vi "WoD Main.vi"() -> ()   [LabVIEW 2017]
uses:
  <vilib>/Platform/TimedLoop/XDataNode/wakeup.ctl
  <vilib>/Platform/TimedLoop/XDataNode/XDNodeRunTimeDep.lvlib
  <vilib>/Platform/TimedLoop/XDataNode/nitl_modes.ctl
  <vilib>/Platform/TimedLoop/XDataNode/timing_clust.ctl
  <vilib>/platform/TimedLoop/XDataNode/XDataNode.xnode
  <vilib>/myRIO/Common/Instrument Driver Framework/myRIO v1.0/DIO/typedefs/DIO Channels Enum.ctl
  <vilib>/myRIO/Common/Instrument Driver Framework/myRIO v1.0/DIO/typedefs/DIO Channels List.ctl
  <vilib>/myRIO/Common/Instrument Driver Framework/Utilities/typedefs/Generic FPGA Reference.ctl
  <vilib>/myRIO/Common/Instrument Driver Framework/Utilities/typedefs/myRIO v1.0 Reference.ctl
  <vilib>/myRIO/Common/Instrument Driver Framework/Utilities/typedefs/Hardware Version Enum.ctl
  <vilib>/myRIO/Common/Instrument Driver Framework/Utilities/typedefs/myRIO Generic Hardware Reference.ctl
  <vilib>/myRIO/Instrument Drivers/Onboard IO/DIO/typedefs/DIO Reference.ctl
  <vilib>/myRIO/Instrument Drivers/Onboard IO/DIO/DIO.lvlib
  <vilib>/myRIO/Instrument Drivers/Onboard IO/DIO/vis/Read.vi
  <vilib>/myRIO/Instrument Drivers/Onboard IO/DIO/vis/myRIO DIO Open.xnode
  <vilib>/myRIO/Common/Instrument Driver Framework/Utilities/vis/Is FPGA Ref Available.vi
  <vilib>/myRIO/Express VI/Onboard IO/DI/DI Express VI.xnode
  <vilib>/myRIO/Common/Instrument Driver Framework/myRIO v1.0/DIO/vis/myRIO v1.1 Open DIO.vi
  <vilib>/userdefined/High Color/nirio_resource_hc.ctl
panel:
  out "Laser Error":errorcluster
  in  "Stop Button":bool
  in  "Select Test":T1(ring)
  in  "Air Bearings?":bool
  in  "Target Speed (rpm)":u32
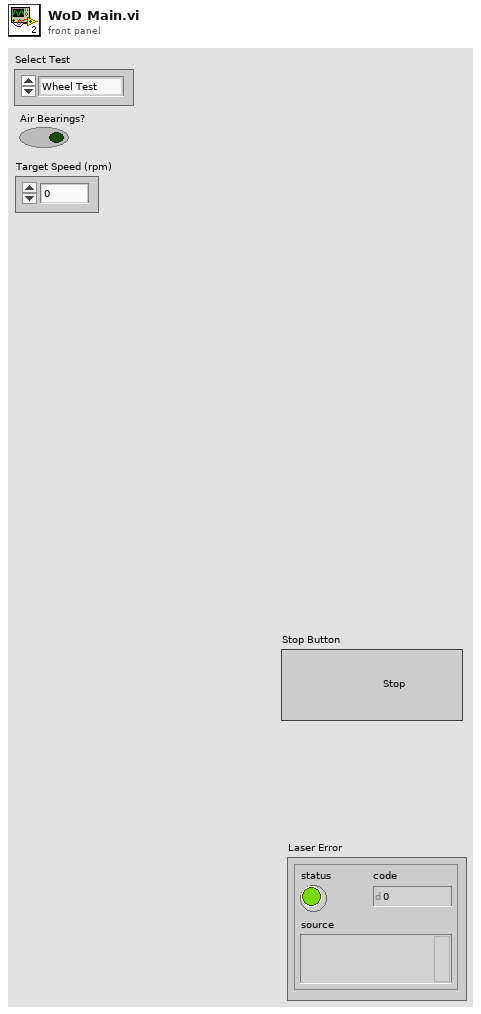
[diagram p1: front panel]
types:
  T1 = enum16{"Wheel Test", "Magnetic Braking Test", "Friction Brake Test", "Material Test", "Air Bearing Test"}
  T2 = typedef "XDNodeRunTimeDep.lvlib/timing_clust.ctl" = cluster{"Expected End [f-1]":u64, "Actual End [f-1]":u64, "Finished Late? [f-1]":bool, "Expected End [i-1]":u64, "Actual End [i-1]":u64, "Finished Late? [i-1]":bool, "Expected Start [i]":u64, "Actual Start [i]":u64, "Expected Start [f]":u64, "Actual Start [f]":u64, "Source Name":string, "Structure Name":string, "Period":i64, "Deadline":i64, "Offset":i64, "Start":i64, "Priority":i32, "Timeout":i32, "Mode":T3, "Wakeup Reason":T4, "Error":errorcluster, "Source Type":string, "Secondary Source Type":string, "Global End Time":u64, "Global Start Time":u64, "Frame Duration":u64, "Iteration Duration":u64, "Assigned CPU":i32, "I/O Scan Engine Mode":u32}
  T3 = typedef "XDNodeRunTimeDep.lvlib/nitl_modes.ctl" = enum32{"No Change", "Process missed periods, maintain original phase", "Discard missed periods, maintain original phase", "Process missed periods, ignore original phase", "Discard missed periods, ignore original phase"}
  T4 = typedef "XDNodeRunTimeDep.lvlib/wakeup.ctl" = enum32{"Normal", "Aborted", "Asynchronous wakeup", "Timing source error", "Timed loop error", "Timeout"}
  T5 = typedef "DIO.lvlib/DIO Reference.ctl" = cluster{"myRIO Reference":T6, "DIO Channels List":T10}
  T6 = typedef "myRIO Generic Hardware Reference.ctl" = cluster{"myRIO Model":T7, "myRIO Hardware Reference":T8}
  T7 = typedef "Hardware Version Enum.ctl" = enum16{"Unknown", "myRIO-1900", "myRIO-1950", "roboRIO", "NI ELVIS RIO CM"}
  T8 = typedef "myRIO v1.0 Reference.ctl" = cluster{"Generic FPGA Reference":T9, "Allow multiple opens":bool}
  T9 = typedef "Generic FPGA Reference.ctl" = refnum<k20>
  T10 = typedef "DIO Channels List.ctl" = T11[]
  T11 = typedef "DIO Channels Enum.ctl" = enum16{"Not Connected", "C/DIO0", "C/DIO1", "C/DIO2", "C/DIO3", "C/DIO4", "C/DIO5", "C/DIO6", "C/DIO7", "A/DIO0", "A/DIO1", "A/DIO2", "A/DIO3", "A/DIO4", "A/DIO5", "A/DIO6", "A/DIO7", "A/DIO8", "A/DIO9", "A/DIO10", "A/DIO11", "A/DIO12", "A/DIO13", "A/DIO14", "A/DIO15", "B/DIO0", "B/DIO1", "B/DIO2", "B/DIO3", "B/DIO4", "B/DIO5", "B/DIO6", "B/DIO7", "B/DIO8", "B/DIO9", "B/DIO10", "B/DIO11", "B/DIO12", "B/DIO13", "B/DIO14", "B/DIO15", "LED0", "LED1", "LED2", "LED3", "Button0", "DIO/DIO0", "DIO/DIO1", "DIO/DIO2", "DIO/DIO3", "DIO/DIO4", "DIO/DIO5", "DIO/DIO6", "DIO/DIO7", "DIO/DIO8", "DIO/DIO9", "SPI/CS0", "SPI/CS1", "SPI/CS2", "SPI/CS3", "LED RADIO (Green)", "LED RADIO (Red)", "LED COMM (Green)", "LED COMM (Red)", "LED MODE (Green)", "LED MODE (Red)"}
  T12 = typedef "nirio_resource_hc.ctl" = tag
  T13 = typedef "allLaserReadings.ctl" = cluster{"Fancy Laser 1":T14, "Fancy Laser 2":T14, "Simple Laser 1":T14, "Simple Laser 2":T14, "Time Stamp":timestamp}
  T14 = typedef "laserReading.ctl" = cluster{"Laser":bool, "Stripe Count":u32, "Last 10 Rising Edges":timestamp[]}
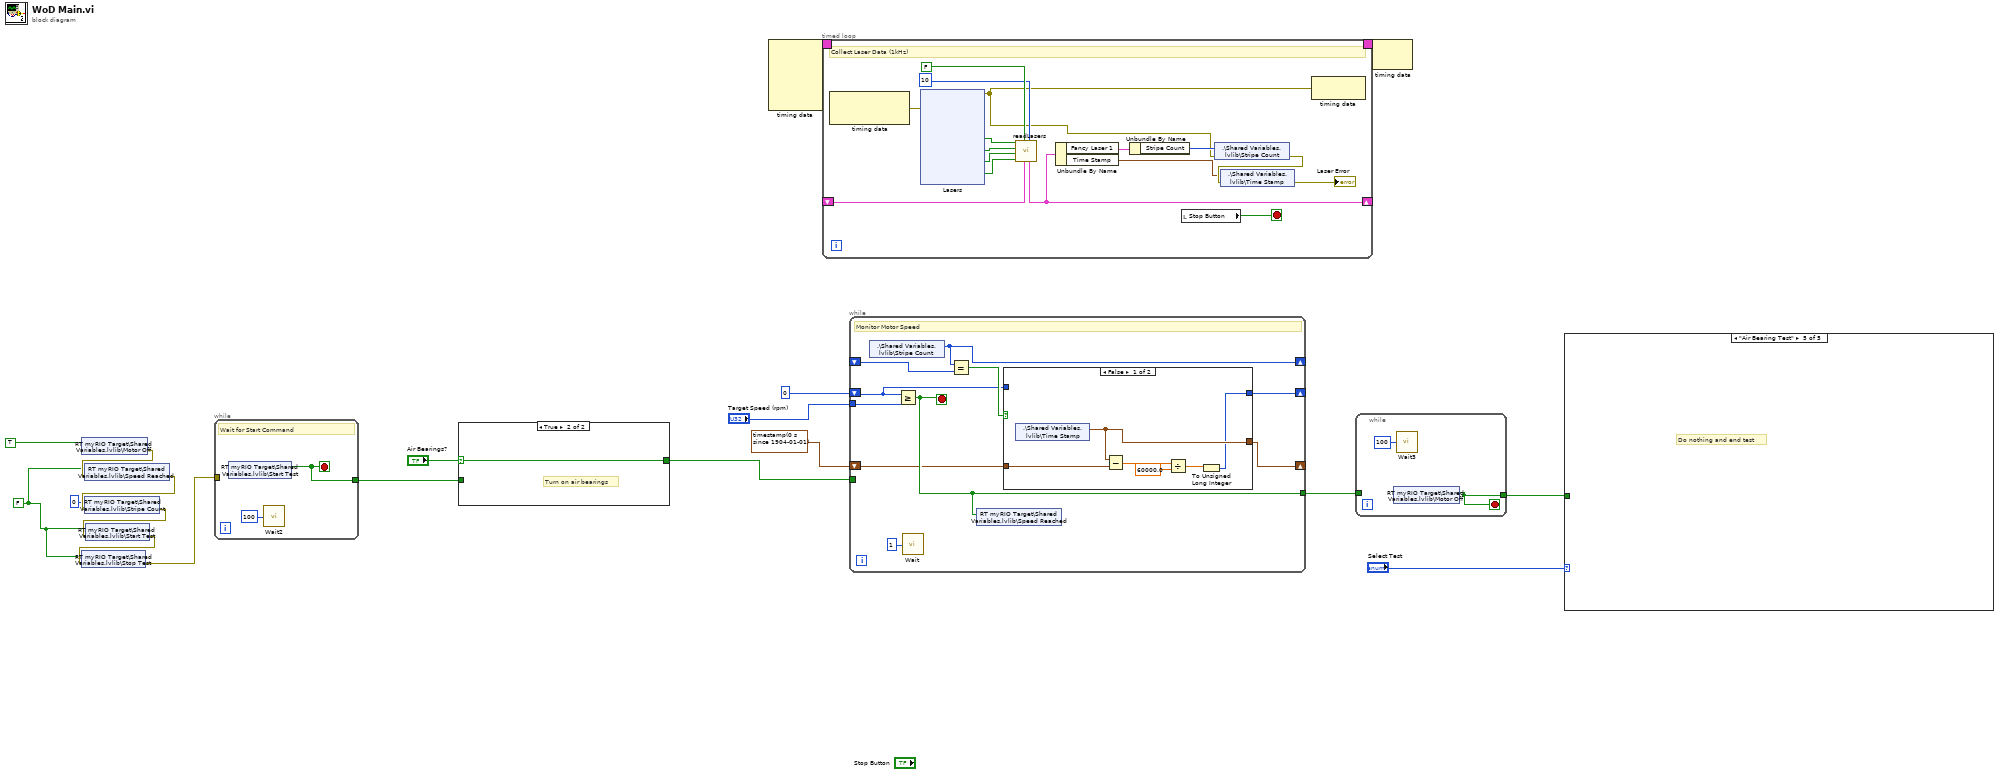
[diagram p0: block diagram]
diagram:
  w3 = FALSE
  n1 = shared-variable "RT myRIO Target\\Shared Variables.lvlib\\Motor Off"(TRUE) -> (error out=w7:errorcluster)  [unwired: 1 in]
  n2 = shared-variable "RT myRIO Target\\Shared Variables.lvlib\\Speed Reached"(w3, error in=w7) -> (error out=w6:errorcluster)
  n3 = shared-variable "RT myRIO Target\\Shared Variables.lvlib\\Stripe Count"(0 ("Stripe Count"), error in=w6) -> (error out=w5:errorcluster)
  n4 = shared-variable "RT myRIO Target\\Shared Variables.lvlib\\Start Test"(w3, error in=w5) -> (error out=w4:errorcluster)
  n5 = shared-variable "RT myRIO Target\\Shared Variables.lvlib\\Stop Test"(w3, error in=w4) -> (error out=w1:errorcluster)
  n6 = while {
    tunnel: [w20] -> w18
    tunnel: w1 -> [_]
    stop <- w20 stop-if-true
    # "Wait for Start Command"
    n7 = shared-variable "RT myRIO Target\\Shared Variables.lvlib\\Start Test"() -> (w20:bool)  [unwired: 1 in, 1 out]
    n8 = call "Wait2"("Count(mSec)"=u32 100) -> ()  [unwired: 1 out]
  }
  n9 = case shown="True" "Air Bearings?" {
    selector: "Air Bearings?" -> [_ w22]
    tunnel: w18 -> [_ _]
    tunnel: [_ w22] -> w17
    frame False {
    }
    frame True {
      # "Turn on air bearings"
    }
  }
  n10 = node-c288() -> (w15:T2)  [unwired: 5 in]
  n11 = timed-loop {
    timing: w15 -> [_]
    timing-out: [_] -> w14
    shift-right: [w29] -> _
    shift-left: _ -> [w32]
    stop <- w38 stop-if-true
    # "Collect Laser Data (1kHz)"
    n12 = node-c288() -> (w37:errorcluster)  [unwired: 1 in, 1 out]
    n13 = xnode "Lasers"("error in (no error)"=w37) -> ("Fancy Laser 1 (B/DIO11 (Pin 18))"=w35:bool, "Fancy Laser 2 (A/DIO7 (Pin 25))"=w33:bool, "Laser 1 (B/DIO9 (Pin 29))"=w36:bool, "Laser 2 (B/DIO10 (Pin 31))"=w34:bool, "error out"=w26:errorcluster)
    n14 = call "readLasers.vi"("Prior Lows"=u8 10, "Laser Readings In"=w32, "Reset Count"=FALSE, "Simple Laser 2"=w34, "Simple Laser 1"=w36, "Fancy Laser 2"=w33, "Fancy Laser 1"=w35) -> ("Laser Readings Out"=w29:T13)  [unwired: 4 in]
    n15 = Unbundle By Name(w29) -> ("Fancy Laser 1"=w28:T14, "Time Stamp"=w23:timestamp)
    n16 = Unbundle By Name(w28) -> ("Stripe Count"=w27:u32)
    n17 = local read "Stop Button"() -> (w38:bool)
    n18 = shared-variable ".\\Shared Variables.lvlib\\Stripe Count"(w27, error in=w26) -> (error out=w25:errorcluster)
    n19 = shared-variable ".\\Shared Variables.lvlib\\Time Stamp"(w23, error in=w25) -> (error out=→"Laser Error":errorcluster)
    n20 = node-c288(w26) -> ()  [unwired: 1 out]
  }
  n21 = while {
    tunnel: w17 -> [_]
    tunnel: "Target Speed (rpm)" -> [w87]
    tunnel: [w86] -> w10
    shift-right: [w89] -> _
    shift-left: _ -> [w90]
    shift-right: [w84] -> _
    shift-left: timestamp(0 s since 1904-01-01) -> [w85]
    shift-right: [w83] -> _
    shift-left: u32 0 ("Target Speed (rpm) 2") -> [w82]
    stop <- w86 stop-if-true
    # "Monitor Motor Speed"
    n22 = shared-variable ".\\Shared Variables.lvlib\\Stripe Count"() -> (w89:i32)  [unwired: 1 in, 1 out]
    n23 = Greater Or Equal?(x=w82, y=w87) -> (x >= y?=w86:bool)
    n24 = call "Wait"("Count(mSec)"=u32 1) -> ()  [unwired: 1 out]
    n25 = Equal?(x=w89, y=w90) -> (x = y?=w88:bool)
    n26 = shared-variable "RT myRIO Target\\Shared Variables.lvlib\\Speed Reached"(w86) -> ()  [unwired: 1 in, 1 out]
    n27 = case shown="False" w88 {
      tunnel: w85 -> [w97 w99]
      tunnel: [w96 w99] -> w84
      tunnel: [w92 w98] -> w83
      tunnel: w82 -> [_ w98]
      frame False {
        n28 = shared-variable ".\\Shared Variables.lvlib\\Time Stamp"() -> (w96:timestamp)  [unwired: 1 in, 1 out]
        n29 = Subtract(x=w96, y=w97) -> (x-y=w95:dbl)
        n30 = Divide(x=w95, y=60000.0) -> (x/y=w93:dbl)
        n31 = To Unsigned Long Integer(number=w93) -> (unsigned 32bit integer=w92:u32)
      }
      frame True {
      }
    }
  }
  n32 = while {
    tunnel: w10 -> [_]
    tunnel: [w100] -> w9
    stop <- w100 stop-if-true
    n33 = shared-variable "RT myRIO Target\\Shared Variables.lvlib\\Motor Off"() -> (w100:bool)  [unwired: 1 in, 1 out]
    n34 = call "Wait3"("Count(mSec)"=u32 100) -> ()  [unwired: 1 out]
  }
  n35 = node-c288(w14) -> ()  [unwired: 1 out]
  n36 = case shown="\"Air Bearing Test\"" "Select Test" {
    tunnel: w9 -> [_ _ _ _ _]
    frame "Material Test", Default {
      # "Do nothing and end test"
    }
    frame "Magnetic Braking Test" {
      # "Trigger relay to move magnetic brake"
    }
    frame "Friction Brake Test" {
      # "Trigger friction brake relay"
    }
    frame "Material Test" {
      # "Do nothing and end test"
    }
    frame "Air Bearing Test" {
      # "Do nothing and end test"
    }
  }
